vi "Configuration Window.vi"(8 "error in (no error)":errorcluster, 11 "Inst.FP":refnum<class "Inst.FP.lvclass">) -> (0 "error out":errorcluster, 3 "Inst.FP":refnum<class "Inst.FP.lvclass">)   [LabVIEW 2019, in "Inst.FP.lvclass"]
uses:
  Inst.FP.lvclass
  Typedefs/Inst.FP.Type--Enum.ctl
  Inst.FP.lvclass/Inst.FP.ctl
  FP-TC-Shared/FP-TC-Shared.lvclass
panel:
  in  "Paths":string
  in  "FP Type":T1
  in  "Cancel":bool
  in  "OK":bool
  # "Confirm or Make Changes:"
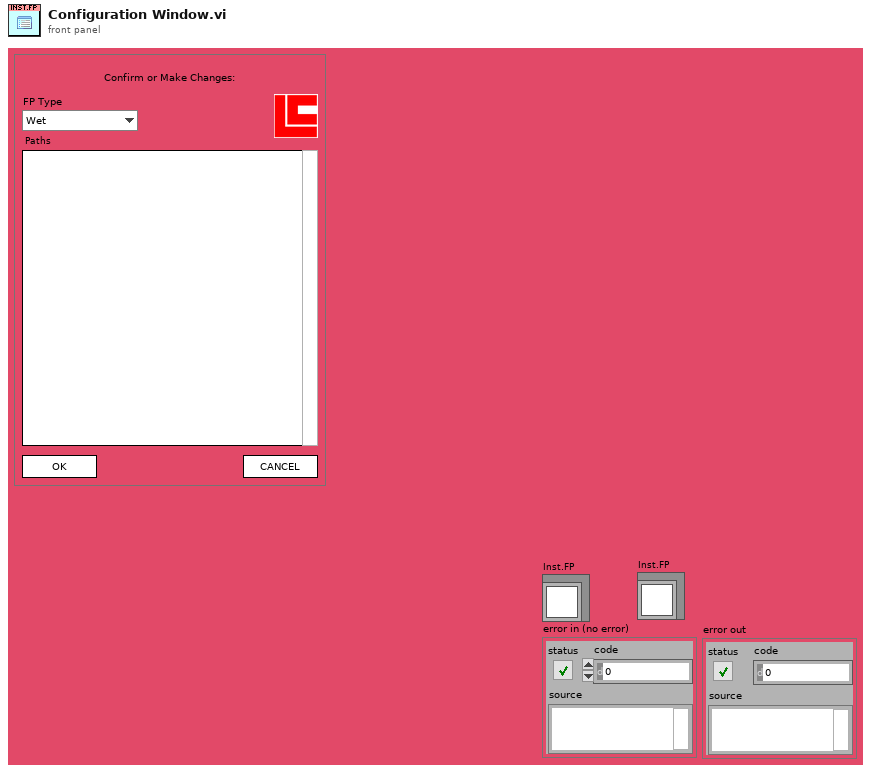
[diagram p1: front panel]
types:
  T1 = typedef "Inst.FP.lvclass/Inst.FP.Type--Enum.ctl" = enum32{"Wet", "CF"}
  T2 = enum32{"Invalid", "Standard", "Closed", "Hidden", "Minimized", "Maximized"}
  T3 = enum32{"invalid app kind", "Development System", "Run Time System", "Student Edition", "Embedded LabVIEW", "Evaluation", "Custom"}
  T4 = cluster{"Core":cluster{"Current VI Reference":refnum<vi>, "Close Panel on Exit?":bool}, "Inst.FP":refnum<class "Inst.FP.lvclass">}
  T5 = cluster{"Current VI Reference":refnum<vi>, "Close Panel on Exit?":bool}
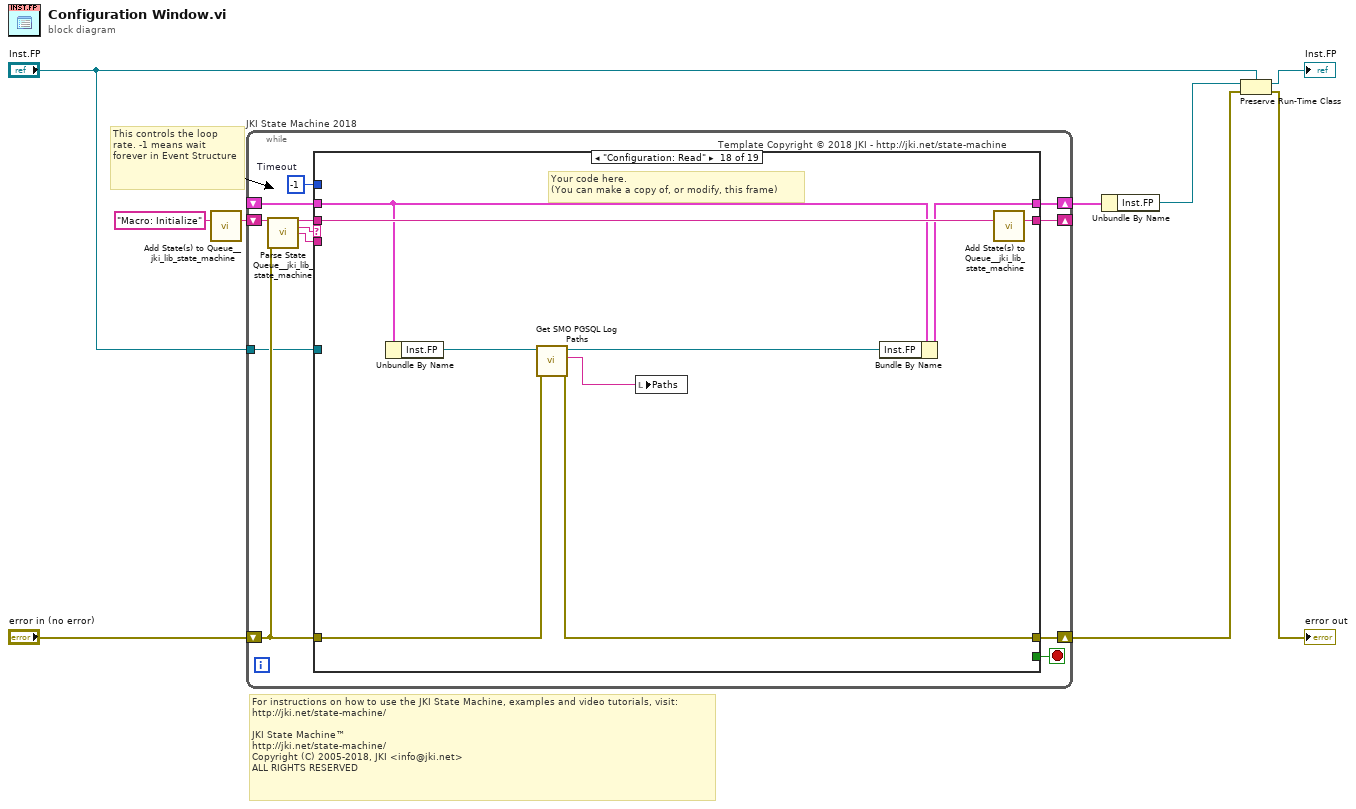
[diagram p0: block diagram]
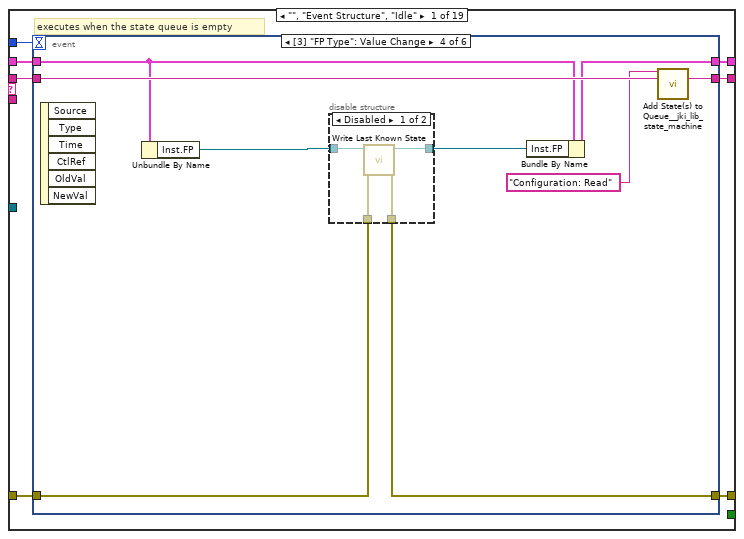
[diagram p2: hidden frame]
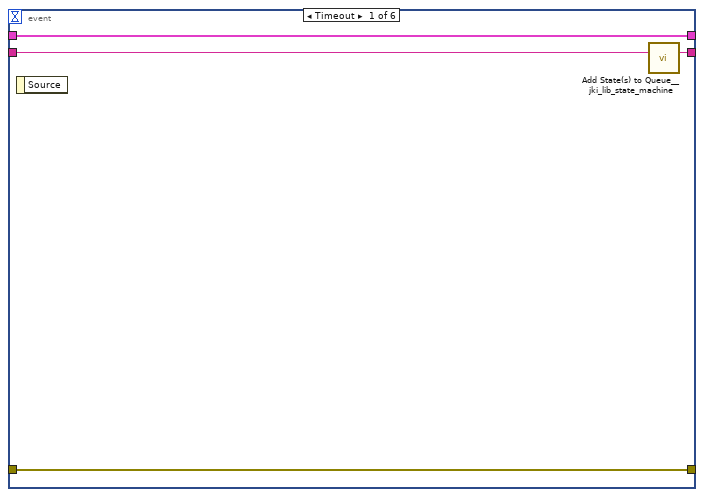
[diagram p3: hidden frame]
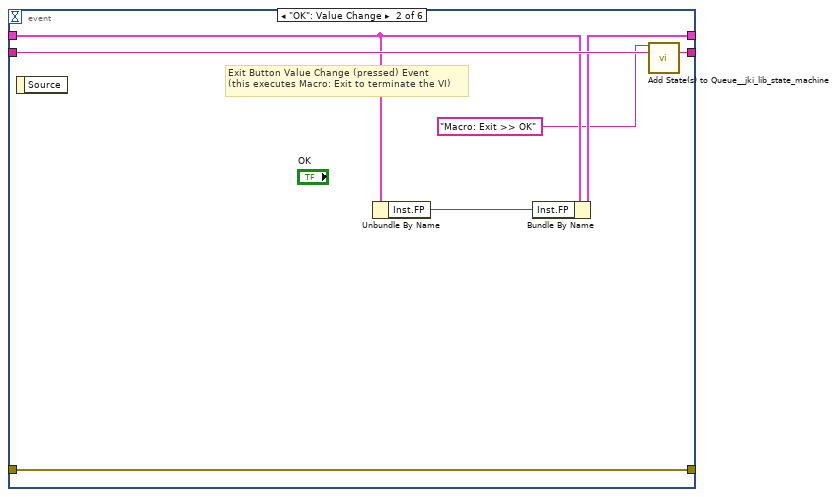
[diagram p4: hidden frame]
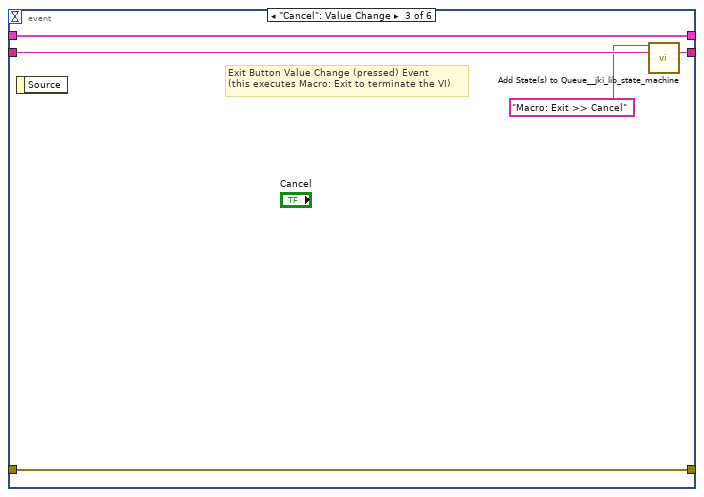
[diagram p5: hidden frame]
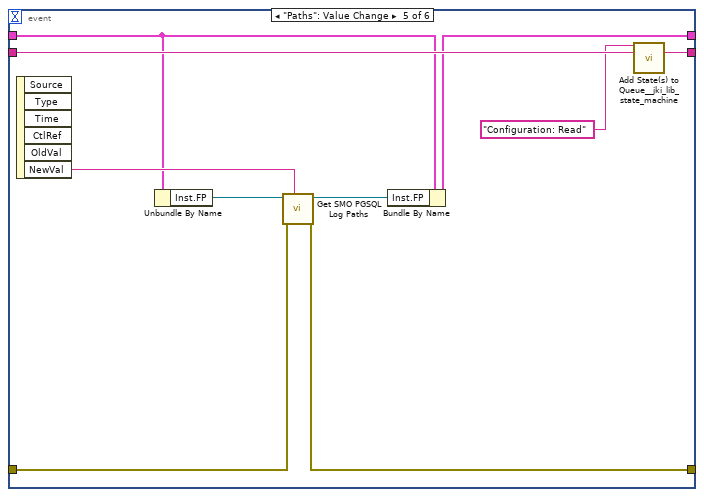
[diagram p7: hidden frame]
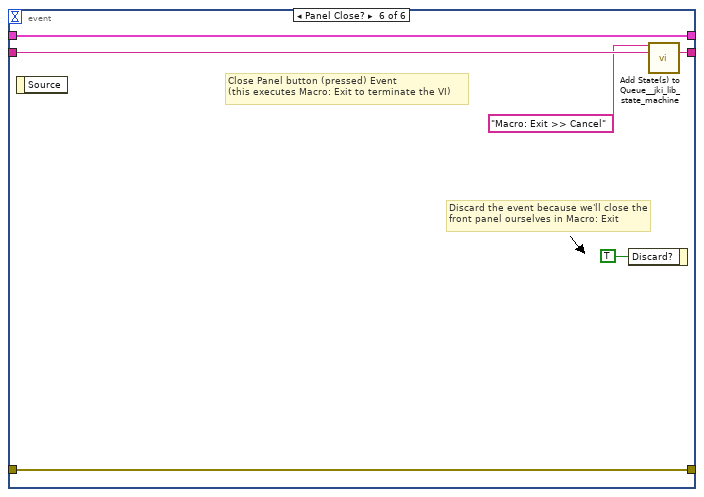
[diagram p8: hidden frame]
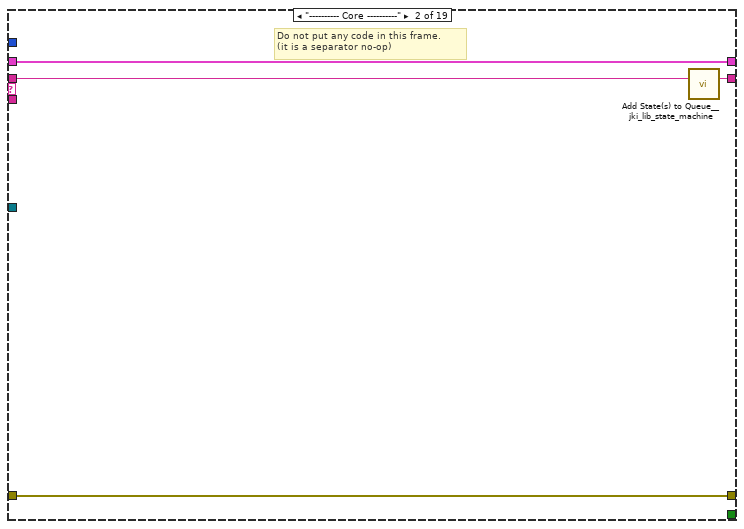
[diagram p9: hidden frame]
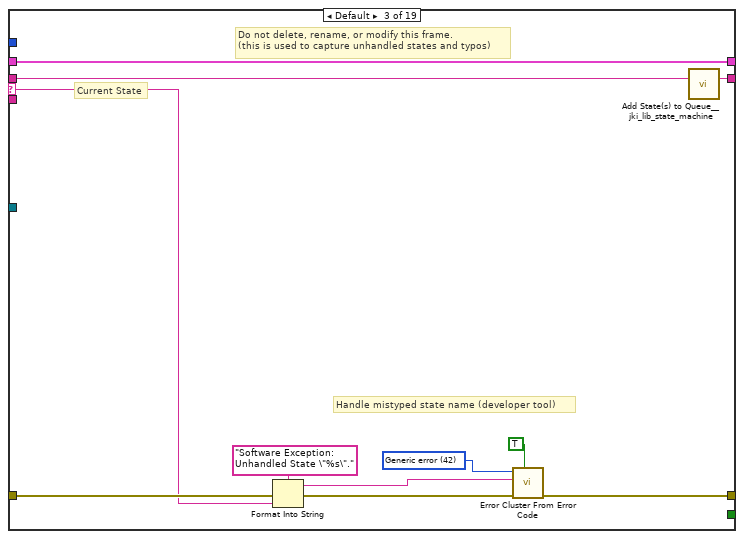
[diagram p10: hidden frame]
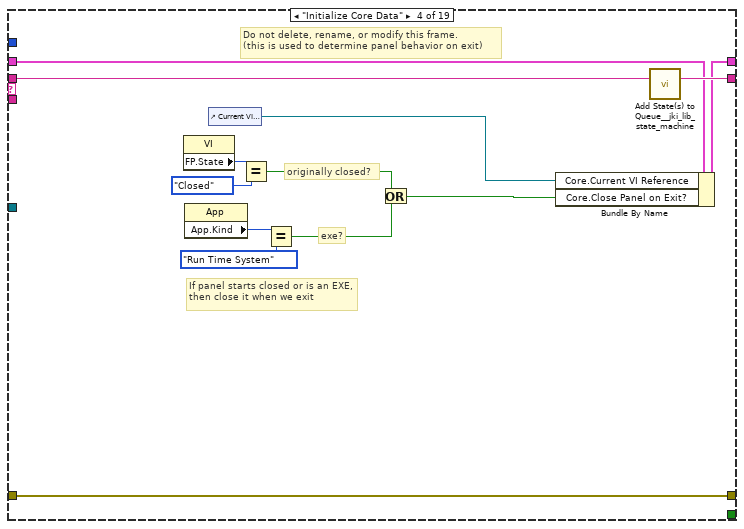
[diagram p11: hidden frame]
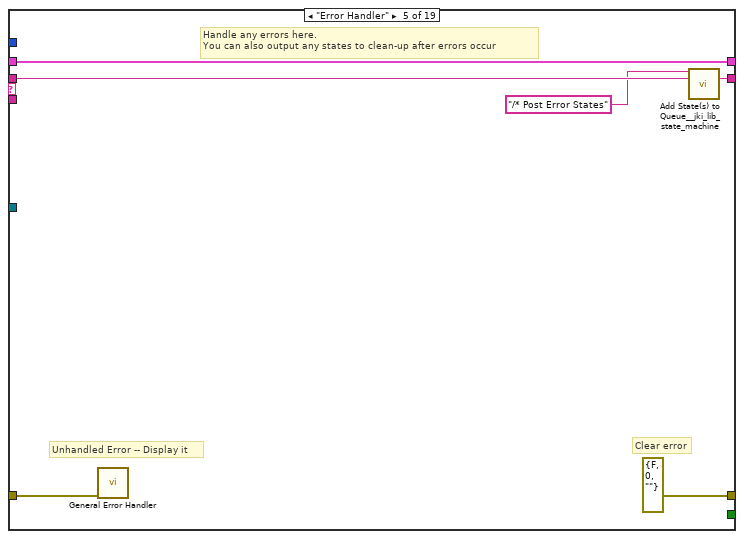
[diagram p12: hidden frame]
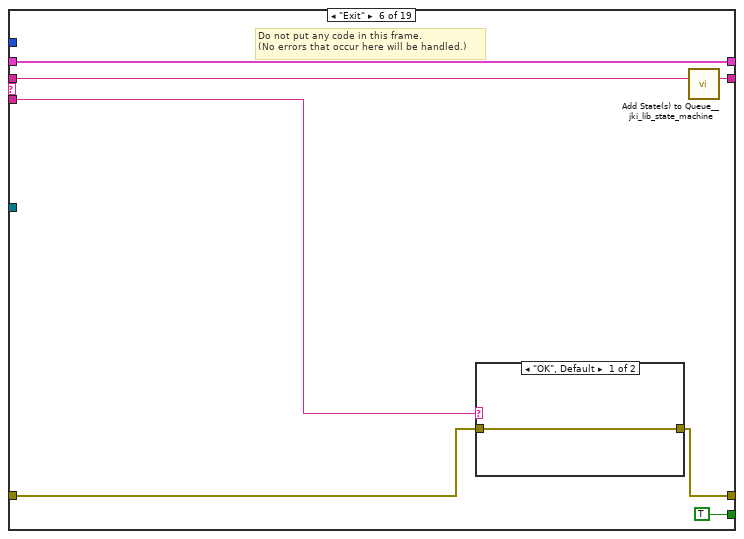
[diagram p13: hidden frame]
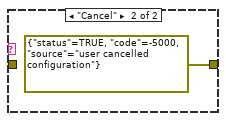
[diagram p14: hidden frame]
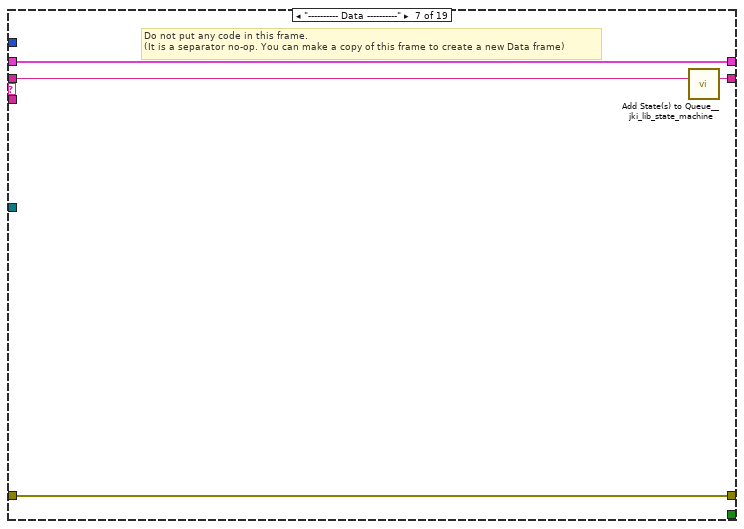
[diagram p15: hidden frame]
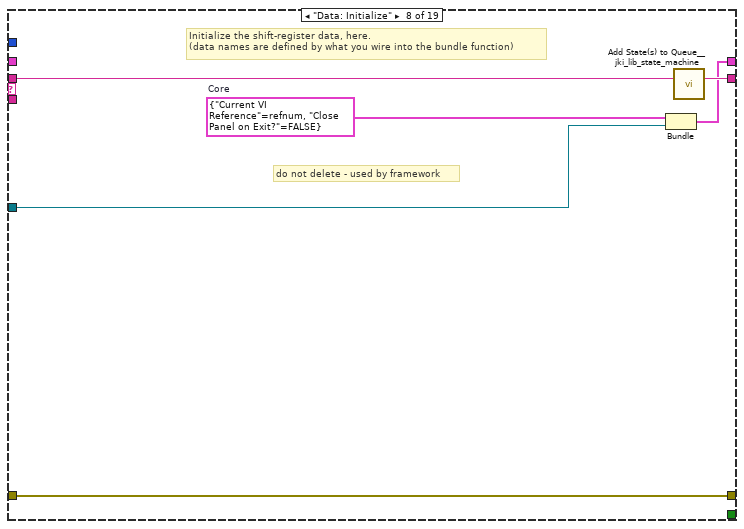
[diagram p16: hidden frame]
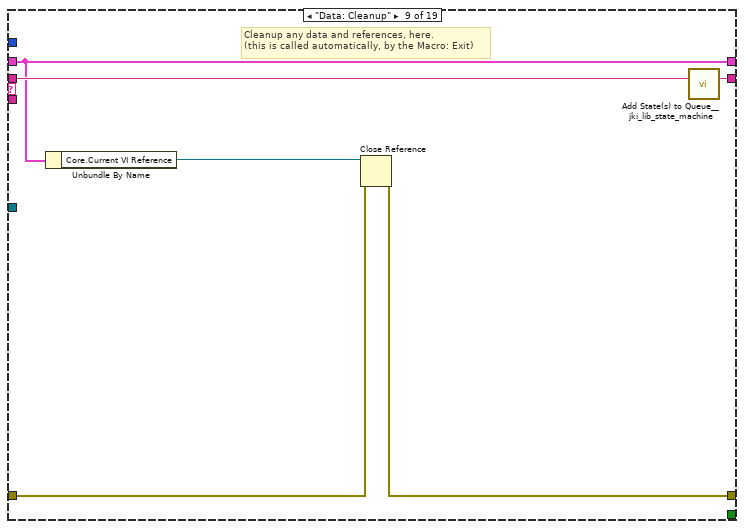
[diagram p17: hidden frame]
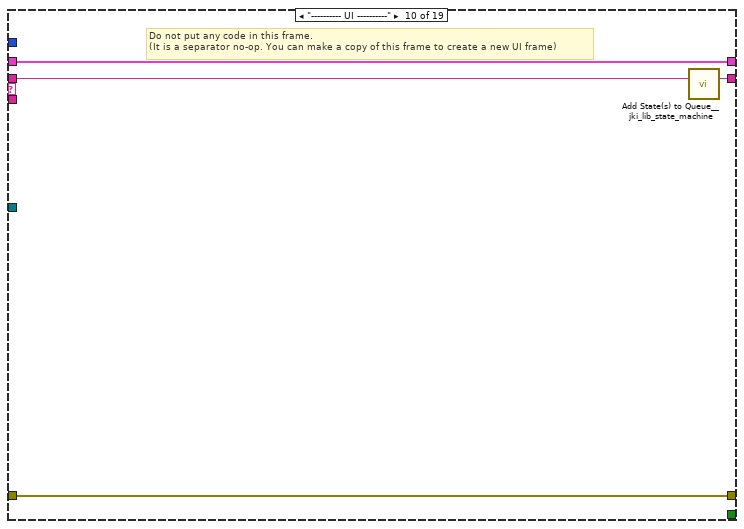
[diagram p18: hidden frame]
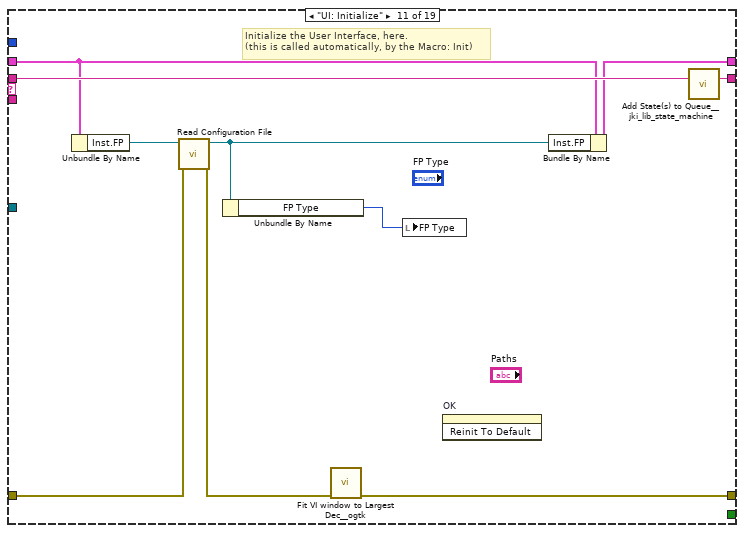
[diagram p19: hidden frame]
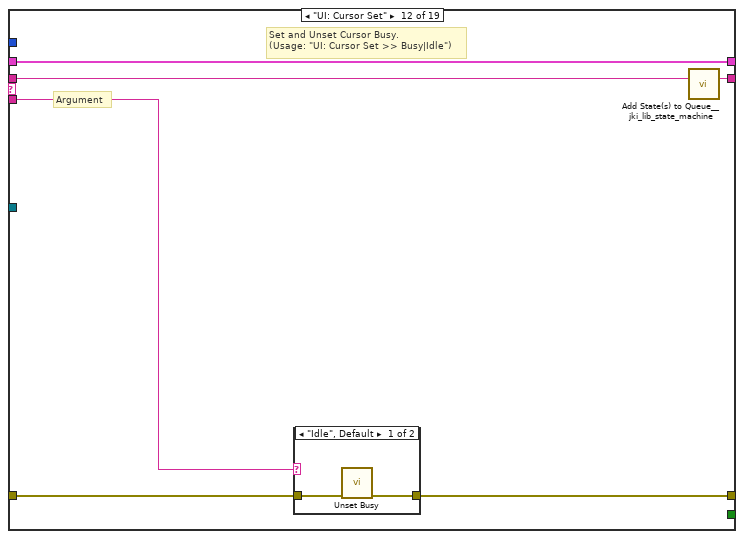
[diagram p20: hidden frame]
diagram:
  # "For instructions on how to use the JKI State Machine, examples and video tutorials, visit:\nhttp://jki.net/state-machine/\n\nJKI State Machine™\nhttp://jki.net/state-machine/\nCopyright (C) 2005-2018, JKI <info@jki.net>\nALL RIGHTS RESERVED"
  # "This controls the loop rate. -1 means wait forever in Event Structure"
  n1 = call <vilib>:"Add State(s) to Queue__jki_lib_state_machine.vi"("State(s) in (\"\")"="Macro: Initialize") -> ("States Out"=w6:string)  [unwired: 14 in]
  n2 = while "JKI State Machine 2018" {
    shift-right: [w14] -> w3
    shift-left: _ -> [w13]
    shift-right: [w17] -> w4
    shift-left: "error in (no error)" -> [w11]
    shift-right: [w16] -> _
    shift-left: w6 -> [w18]
    tunnel: "Inst.FP" -> [w10]
    stop <- w15 stop-if-true
    w12 = -1  # Timeout
    # "Template Copyright © 2018 JKI - http://jki.net/state-machine"
    n3 = call <vilib>:"Parse State Queue__jki_lib_state_machine.vi"("State Queue"=w18, "Error In (no error)"=w11) -> ("Remaining States"=w20:string, "Current State"=w21:string, "Arguments"=w19:string)  [unwired: 11 in]
    n4 = case shown="\"Configuration: Read\"" w21 {
      selector: w21 -> [_ _ w79 _ _ _ _ _ _ _ _ _ _ _ _ _ _ _ _]
      tunnel: w20 -> [w28 w78 w83 w102 w108 w115 w121 w127 w133 w137 w147 w153 w164 w233 w238 w253 w257 w266 w272]
      tunnel: w19 -> [_ _ _ _ _ w111 _ _ _ _ _ w148 w158 _ _ w242 _ _ _]
      tunnel: w13 -> [w26 w75 w81 w95 w105 w113 w118 _ w128 w134 w144 w151 w160 w230 w235 w250 w254 w263 w268]
      tunnel: [w25 w76 w85 w99 errorcluster {"status"=FALSE, "code"=0, "source"=""} ("error out") w109 w119 w123 w129 w135 w145 w149 w161 w231 w236 w251 w255 w261 w269] -> w17
      tunnel: w11 -> [w24 w76 w84 w99 w104 w110 w119 w123 w130 w135 w141 w150 w162 w231 w236 w251 w255 w262 w269]
      tunnel: [w27 w77 w82 w101 w107 w114 w120 w126 w132 w136 w146 w152 w163 w232 w237 w252 w256 w265 w271] -> w16
      tunnel: [_ _ _ _ _ TRUE _ _ _ _ _ _ _ _ _ _ _ _ _] -> w15
      tunnel: [w23 w75 w81 w100 w105 w113 w118 w125 w128 w134 w143 w151 w160 w230 w235 w250 w254 w264 w270] -> w14
      tunnel: w12 -> [w22 _ _ _ _ _ _ _ _ _ _ _ _ _ _ _ _ _ _]
      tunnel: w10 -> [_ _ _ _ _ _ _ w122 _ _ _ _ _ _ _ _ _ _ _]
      frame "", "Event Structure", "Idle" {
        # "executes when the state queue is empty"
        n5 = event shown="[3] \"FP Type\": Value Change" {
          selector: _ -> [_ _ _ _ _ _]
          dyn-events: _ -> [_ _ _ _ _ _]
          timeout: w22 -> [_ _ _ _ _ _]
          tunnel: w28 -> [w32 w39 w44 w52 w67 w74]
          tunnel: [w31 w38 w43 w53 w68 w73] -> w27
          tunnel: w26 -> [w29 w35 w40 w49 w59 w71]
          tunnel: [w30 w37 w42 w47 w63 w72] -> w25
          tunnel: w24 -> [w30 w37 w42 w48 w62 w72]
          tunnel: [w29 w36 w40 w50 w60 w71] -> w23
          event Timeout {
            n6 = event-data() -> ()  [unwired: 1 in, 1 out]
            n7 = call <vilib>:"Add State(s) to Queue__jki_lib_state_machine.vi"("State(s) in (\"\")"=w32) -> ("States Out"=w31:string)  [unwired: 14 in]
          }
          event "OK": Value Change {
            # "Exit Button Value Change (pressed) Event\n(this executes Macro: Exit to terminate the VI)"
            n8 = event-data() -> ()  [unwired: 1 in, 1 out]
            n9 = Unbundle By Name(w35) -> ("Inst.FP"=w33:refnum<class "Inst.FP.lvclass">)
            n10 = Bundle By Name(cluster=w35, "Inst.FP"=w33) -> (w36:T4)
            n11 = call <vilib>:"Add State(s) to Queue__jki_lib_state_machine.vi"("State(s) in Front (\"\")"="Macro: Exit >> OK", "State(s) in (\"\")"=w39) -> ("States Out"=w38:string)  [unwired: 13 in]
          }
          event "Cancel": Value Change {
            # "Exit Button Value Change (pressed) Event\n(this executes Macro: Exit to terminate the VI)"
            n12 = event-data() -> ()  [unwired: 1 in, 1 out]
            n13 = call <vilib>:"Add State(s) to Queue__jki_lib_state_machine.vi"("State(s) in Front (\"\")"="Macro: Exit >> Cancel", "State(s) in (\"\")"=w44) -> ("States Out"=w43:string)  [unwired: 13 in]
          }
          event Value Change {
            n14 = event-data() -> ()  [unwired: 1 in, 6 out]
            n15 = Unbundle By Name(w49) -> ("Inst.FP"=w45:refnum<class "Inst.FP.lvclass">)
            n16 = disable-structure shown="Disabled" {
              disable-tunnel: w48 -> [w57 _]
              disable-tunnel: [w56 _] -> w47
              disable-tunnel: [w55 w58] -> w46
              disable-tunnel: w45 -> [w54 w58]
              frame Disabled {
                n17 = call "Write Last Known State.vi"("error in (no error)"=w57, "FP-TC-Shared in"=w54) -> ("error out"=w56:errorcluster, "FP-TC-Shared out"=w55:refnum<class "FP-TC-Shared.lvclass">)  [unwired: 8 in]
              }
              frame Enabled {
              }
            }
            n18 = Bundle By Name(cluster=w49, "Inst.FP"=w46) -> (w50:T4)
            n19 = call <vilib>:"Add State(s) to Queue__jki_lib_state_machine.vi"("State(s) in Front (\"\")"="Configuration: Read" ("State(s) in Front (\"\")"), "State(s) in (\"\")"=w52) -> ("States Out"=w53:string)  [unwired: 13 in]
          }
          event "Paths": Value Change {
            n20 = event-data() -> ("NewVal"=w64:string)  [unwired: 1 in, 5 out]
            n21 = Unbundle By Name(w59) -> ("Inst.FP"=w65:refnum<class "Inst.FP.lvclass">)
            n22 = call-dynamic "Get SMO PGSQL Log Paths.vi"("Paths"=w64, "error in (no error)"=w62, "Inst.FP in"=w65) -> ("error out"=w63:errorcluster, "Inst.FP out"=w61:refnum<class "Inst.FP.lvclass">)  [unwired: 6 in, 1 out]
            n23 = Bundle By Name(cluster=w59, "Inst.FP"=w61) -> (w60:T4)
            n24 = call <vilib>:"Add State(s) to Queue__jki_lib_state_machine.vi"("State(s) in Front (\"\")"="Configuration: Read" ("State(s) in Front (\"\")"), "State(s) in (\"\")"=w67) -> ("States Out"=w68:string)  [unwired: 13 in]
          }
          event Panel Close? {
            # "Discard the event because we'll close the front panel ourselves in Macro: Exit"
            # "Close Panel button (pressed) Event\n(this executes Macro: Exit to terminate the VI)"
            n25 = event-data() -> ()  [unwired: 1 in, 1 out]
            n26 = event-data("Discard?"=TRUE) -> ()  [unwired: 1 in, 1 out]
            n27 = call <vilib>:"Add State(s) to Queue__jki_lib_state_machine.vi"("State(s) in Front (\"\")"="Macro: Exit >> Cancel", "State(s) in (\"\")"=w74) -> ("States Out"=w73:string)  [unwired: 13 in]
          }
        }
      }
      frame "---------- Core ----------" {
        # "Do not put any code in this frame.\n(it is a separator no-op)"
        n28 = call <vilib>:"Add State(s) to Queue__jki_lib_state_machine.vi"("State(s) in (\"\")"=w78) -> ("States Out"=w77:string)  [unwired: 14 in]
      }
      frame Default {
        w88 = 42 items=["No error", "Argument error", "Memory is full", "Out of zone", "End of file", "File already open", "Generic file I/O error", "File not found", "File permission error", "Disk is full", "Duplicate path", "Too many files open", "System feature not enabled", "Resource file not found", "Cannot add resource", "Resource not found", "Image not found", "Image memory error", "Pen does not exist", "Config type invalid", "Config token not found", "Config parse error", "Config memory error", "Bad external code format", "Bad external code offset", "External code not present", "Null window", "Destroy window error", "Null menu", "Print aborted", "Bad print record", "Print driver error", "Windows error during printing", "Memory error during printing", "Print dialog error", "Generic print error", "Invalid device refnum", "Device not found", "Device parameter error", "Device unit error", "Cannot open device", "Device call aborted", "Generic error", "Cancelled by user", "Object ID too low", "Object ID too high", "Object not in heap", "Unknown heap", "Unknown object (invalid DefProc)", "Unknown object (DefProc not in table)", "Message out of range", "Invalid (null) method", "Unknown message", "Manager call not supported", "Bad address", "Network operation in progress", "Network operation timed out", "Connection is busy", "Network attribute not supported", "Network error", "Address in use", "System out of memory", "Connection aborted", "Connection refused", "Not connected", "Already connected", "Connection closed", "Initialization error (interapplication manager)", "Bad occurrence", "Wait on unbound occurrence handler", "Occurrence queue overflow", "Datalog type conflict", "Unused", "Unrecognized type (interapplication manager)", "Memory corrupt", "Failed to make temporary DLL", "Old CIN version", "Drag socket not found", "Failed to load drop-object", "Failed to register OLE object", "Failed to release OLE object", "Format specifier type mismatch", "Unknown format specifier", "Too few format specifiers", "Too many format specifiers", "Scan failed", "Newer CIN version", "Error converting to variant", "Runtime menu error", "Password tampered", "Variant attribute not found", "Incompatible variant data type", "Event data is not available", "Event Store is not present", "Occurrence is not found", "Event Queue is not created", "Event info is not available", "Refnum passed is NULL", "Error retrieving Class GUID", "Error retrieving CoClass GUID", "Error retrieving TypeLib GUID.", "Bad built application magic bytes.", "Specific driver is different from the specific driver associated with the Logical Name.", "There is no session opened to the class driver.", "Max Error", "MAX - Error with config objects", "MAX - Error loading configuration", "MAX - Group not supported"]
        # "Current State"
        # "Do not delete, rename, or modify this frame.\n(this is used to capture unhandled states and typos)"
        # "Handle mistyped state name (developer tool)"
        n29 = Format Into String(format string="Software Exception: Unhandled State \"%s\"." ("message"), error in=w84, w79) -> (resulting string=w87:string, error out=w86:errorcluster)  [unwired: 1 in]
        n30 = call <vilib>:"Error Cluster From Error Code.vi"("show call chain? (False)"=TRUE, "error in (no error)"=w86, "error message (\"\")"=w87, "error code (0)"=w88) -> ("error out"=w85:errorcluster)  [unwired: 5 in]
        n31 = call <vilib>:"Add State(s) to Queue__jki_lib_state_machine.vi"("State(s) in (\"\")"=w83) -> ("States Out"=w82:string)  [unwired: 14 in]
      }
      frame "Initialize Core Data" {
        # "Do not delete, rename, or modify this frame.\n(this is used to determine panel behavior on exit)"
        # "originally closed?"
        # "exe?"
        # "If panel starts closed or is an EXE, then close it when we exit"
        n32 = property class="VI"() -> ("FP.State"=w92:T2)  [unwired: 2 in, 2 out]
        n33 = property class="App"() -> ("App.Kind"=w98:T3)  [unwired: 2 in, 2 out]
        n34 = control-ref of="Current VI Reference"() -> (w93:refnum<vi>)
        n35 = Equal?(x=w92, y=T2."Closed" ("Front Panel Window:State")) -> (x = y?=w90:bool)
        n36 = Equal?(x=w98, y=T3."Run Time System" ("Application:Kind")) -> (x = y?=w96:bool)
        n37 = Or(x=w90, y=w96) -> (x .or. y?=w94:bool)
        n38 = Bundle By Name(cluster=w95, "Core.Current VI Reference"=w93, "Core.Close Panel on Exit?"=w94) -> (w100:T4)
        n39 = call <vilib>:"Add State(s) to Queue__jki_lib_state_machine.vi"("State(s) in (\"\")"=w102) -> ("States Out"=w101:string)  [unwired: 14 in]
      }
      frame "Error Handler" {
        # "Unhandled Error -- Display it"
        # "Handle any errors here.\nYou can also output any states to clean-up after errors occur"
        # "Clear error"
        n40 = call <vilib>:"General Error Handler.vi"("error in (no error)"=w104) -> ()  [unwired: 10 in, 5 out]
        n41 = call <vilib>:"Add State(s) to Queue__jki_lib_state_machine.vi"("State(s) in Front (\"\")"="/* Post Error States", "State(s) in (\"\")"=w108) -> ("States Out"=w107:string)  [unwired: 13 in]
      }
      frame "Exit" {
        # "Do not put any code in this frame.\n(No errors that occur here will be handled.)"
        n42 = case shown="\"OK\", Default" w111 {
          tunnel: w110 -> [w116 _]
          tunnel: [w116 errorcluster {"status"=TRUE, "code"=-5000, "source"="user cancelled configuration"} ("error in (no error)")] -> w109
          frame "OK", Default {
          }
          frame "Cancel" {
          }
        }
        n43 = call <vilib>:"Add State(s) to Queue__jki_lib_state_machine.vi"("State(s) in (\"\")"=w115) -> ("States Out"=w114:string)  [unwired: 14 in]
      }
      frame "---------- Data ----------" {
        # "Do not put any code in this frame.\n(It is a separator no-op. You can make a copy of this frame to create a new Data frame)"
        n44 = call <vilib>:"Add State(s) to Queue__jki_lib_state_machine.vi"("State(s) in (\"\")"=w121) -> ("States Out"=w120:string)  [unwired: 14 in]
      }
      frame "Data: Initialize" {
        w124 = T5 {"Current VI Reference"=refnum, "Close Panel on Exit?"=FALSE}  # Core
        # "do not delete - used by framework"
        # "Initialize the shift-register data, here.\n(data names are defined by what you wire into the bundle function)"
        n45 = Bundle("Core"=w124, "Inst.FP"=w122) -> (w125:T4)  [unwired: 1 in]
        n46 = call <vilib>:"Add State(s) to Queue__jki_lib_state_machine.vi"("State(s) in (\"\")"=w127) -> ("States Out"=w126:string)  [unwired: 14 in]
      }
      frame "Data: Cleanup" {
        # "Cleanup any data and references, here.\n(this is called automatically, by the Macro: Exit)"
        n47 = Unbundle By Name(w128) -> ("Core.Current VI Reference"=w131:refnum<vi>)
        n48 = Close Reference(reference=w131, error in (no error)=w130) -> (error out=w129:errorcluster)
        n49 = call <vilib>:"Add State(s) to Queue__jki_lib_state_machine.vi"("State(s) in (\"\")"=w133) -> ("States Out"=w132:string)  [unwired: 14 in]
      }
      frame "---------- UI ----------" {
        # "Do not put any code in this frame.\n(It is a separator no-op. You can make a copy of this frame to create a new UI frame)"
        n50 = call <vilib>:"Add State(s) to Queue__jki_lib_state_machine.vi"("State(s) in (\"\")"=w137) -> ("States Out"=w136:string)  [unwired: 14 in]
      }
      frame "UI: Initialize" {
        # "Initialize the User Interface, here.\n(this is called automatically, by the Macro: Init)"
        n51 = Unbundle By Name(w144) -> ("Inst.FP"=w140:refnum<class "Inst.FP.lvclass">)
        n52 = call-dynamic "Read Configuration File.vi"("error in (no error)"=w141, "Inst.FP in"=w140) -> ("error out"=w142:errorcluster, "Inst.FP out"=w139:refnum<class "Inst.FP.lvclass">)  [unwired: 8 in]
        n53 = Unbundle By Name(w139) -> ("FP Type"=w138:T1)
        n54 = call <userlib>:"Fit VI window to Largest Dec__ogtk.vi"("error in (no error)"=w142) -> ("error out"=w145:errorcluster)  [unwired: 5 in, 1 out]
        n55 = local write "FP Type"(w138) -> ()
        n56 = invoke on="OK" class="Bool" method="Reinit To Default"() -> ()  [unwired: 3 in, 3 out]
        n57 = Bundle By Name(cluster=w144, "Inst.FP"=w139) -> (w143:T4)
        n58 = call <vilib>:"Add State(s) to Queue__jki_lib_state_machine.vi"("State(s) in (\"\")"=w147) -> ("States Out"=w146:string)  [unwired: 14 in]
      }
      frame "UI: Cursor Set" {
        # "Argument"
        # "Set and Unset Cursor Busy.\n(Usage: \"UI: Cursor Set >> Busy|Idle\")"
        n59 = case shown="\"Idle\", Default" w148 {
          tunnel: w150 -> [w155 w157]
          tunnel: [w154 w156] -> w149
          frame "Idle", Default {
            n60 = call <vilib>:"Unset Busy.vi"("error in (no error)"=w155) -> ("error out"=w154:errorcluster)  [unwired: 10 in]
          }
          frame "Busy" {
            n61 = call <vilib>:"Set Busy.vi"("error in (no error)"=w157) -> ("error out"=w156:errorcluster)  [unwired: 9 in, 1 out]
          }
        }
        n62 = call <vilib>:"Add State(s) to Queue__jki_lib_state_machine.vi"("State(s) in (\"\")"=w153) -> ("States Out"=w152:string)  [unwired: 14 in]
      }
      frame "UI: Front Panel State" {
        # "Argument"
        # "Set Front Panel Open or Closed\n(Usage: \"UI: Front Panel State >> Open|Close\")"
        n63 = Unbundle By Name(w160) -> ("Core.Current VI Reference"=w159:refnum<vi>)
        n64 = case shown="\"Open\", \"Standard\", Default" w158 {
          tunnel: w162 -> [w170 w185 w196 w209 w222]
          tunnel: [w172 w186 w198 w211 w224] -> w161
          tunnel: w159 -> [w171 w183 w197 w210 w223]
          frame "Open", "Standard", Default {
            w165 = T2."Standard" ("State")
            n65 = property class="VI"(reference=w171, error in=w170) -> (reference out=w168:refnum<vi>, error out=w169:errorcluster, "FP.State"=w167:T2)
            n66 = Not Equal?(x=w167, y=w165) -> (x != y?=w166:bool)
            n67 = case shown="False" w166 {
              tunnel: [w176 w178] -> w172
              tunnel: w169 -> [w175 w178]
              tunnel: w168 -> [w174 _]
              tunnel: w165 -> [w173 _]
              frame True {
                n68 = invoke class="VI" method="FP.Open"(reference=w174, error in=w175, "Activate"=TRUE, "State"=w173) -> (error out=w176:errorcluster)  [unwired: 1 in, 4 out]
              }
              frame False {
              }
            }
          }
          frame "Close", "Closed" {
            n69 = property class="VI"(reference=w183, error in=w185) -> (reference out=w182:refnum<vi>, error out=w184:errorcluster, "FP.State"=w180:T2)
            n70 = Not Equal?(x=w180, y=T2."Closed" ("Front Panel Window:State")) -> (x != y?=w179:bool)
            n71 = case shown="True" w179 {
              tunnel: [w187 w190] -> w186
              tunnel: w184 -> [w187 w189]
              tunnel: w182 -> [_ w188]
              frame False {
              }
              frame True {
                n72 = invoke class="VI" method="FP.Close"(reference=w188, error in=w189) -> (error out=w190:errorcluster)  [unwired: 1 in, 2 out]
              }
            }
          }
          frame "Hidden", "Hide" {
            w191 = T2."Hidden" ("State")
            n73 = property class="VI"(reference=w197, error in=w196) -> (reference out=w194:refnum<vi>, error out=w195:errorcluster, "FP.State"=w193:T2)
            n74 = Not Equal?(x=w193, y=w191) -> (x != y?=w192:bool)
            n75 = case shown="True" w192 {
              tunnel: [w202 w203] -> w198
              tunnel: w195 -> [w201 w203]
              tunnel: w194 -> [w200 _]
              tunnel: w191 -> [w199 _]
              frame True {
                n76 = invoke class="VI" method="FP.Open"(reference=w200, error in=w201, "State"=w199) -> (error out=w202:errorcluster)  [unwired: 2 in, 4 out]
              }
              frame False {
              }
            }
          }
          frame "Minimize", "Minimized" {
            w204 = T2."Minimized" ("State")
            n77 = property class="VI"(reference=w210, error in=w209) -> (reference out=w207:refnum<vi>, error out=w208:errorcluster, "FP.State"=w206:T2)
            n78 = Not Equal?(x=w206, y=w204) -> (x != y?=w205:bool)
            n79 = case shown="True" w205 {
              tunnel: [w215 w216] -> w211
              tunnel: w208 -> [w214 w216]
              tunnel: w207 -> [w213 _]
              tunnel: w204 -> [w212 _]
              frame True {
                n80 = invoke class="VI" method="FP.Open"(reference=w213, error in=w214, "State"=w212) -> (error out=w215:errorcluster)  [unwired: 2 in, 4 out]
              }
              frame False {
              }
            }
          }
          frame "Maximize", "Maximized" {
            w217 = T2."Maximized" ("State")
            n81 = property class="VI"(reference=w223, error in=w222) -> (reference out=w220:refnum<vi>, error out=w221:errorcluster, "FP.State"=w219:T2)
            n82 = Not Equal?(x=w219, y=w217) -> (x != y?=w218:bool)
            n83 = case shown="True" w218 {
              tunnel: [w228 w229] -> w224
              tunnel: w221 -> [w227 w229]
              tunnel: w220 -> [w226 _]
              tunnel: w217 -> [w225 _]
              frame True {
                n84 = invoke class="VI" method="FP.Open"(reference=w226, error in=w227, "State"=w225) -> (error out=w228:errorcluster)  [unwired: 2 in, 4 out]
              }
              frame False {
              }
            }
          }
        }
        n85 = call <vilib>:"Add State(s) to Queue__jki_lib_state_machine.vi"("State(s) in (\"\")"=w164) -> ("States Out"=w163:string)  [unwired: 14 in]
      }
      frame "---------- Macro ----------" {
        # "Do not put any code in this frame.\n(It is a separator no-op. You can make a copy of this frame to create a new Macro frame)"
        n86 = call <vilib>:"Add State(s) to Queue__jki_lib_state_machine.vi"("State(s) in (\"\")"=w233) -> ("States Out"=w232:string)  [unwired: 14 in]
      }
      frame "Macro: Initialize" {
        w234 = "Data: Initialize\nInitialize Core Data\nUI: Initialize\nUI: Front Panel State >> Open\nConfiguration: Read"  # Data: Initialize Initialize Core Data UI: Initialize UI: Front Panel State >> Open Configuration: Read
        # "Initialization Macro\n(This is called once, when the VI starts)"
        n87 = call <vilib>:"Add State(s) to Queue__jki_lib_state_machine.vi"("State(s) in Front (\"\")"=w234, "State(s) in (\"\")"=w238) -> ("States Out"=w237:string)  [unwired: 13 in]
      }
      frame "Macro: Exit" {
        # "Exit Macro\n(This is called once, when the VI exits)"
        n88 = Unbundle By Name(w250) -> ("Core.Close Panel on Exit?"=w249:bool)
        n89 = call <vilib>:"Build State String with Arguments__JKI_lib_State_Machine.vi"("Arguments (\"\")"=w242, "State"="Exit") -> ("State with Arguments"=w240:string)  [unwired: 4 in]
        n90 = Select(t="UI: Front Panel State >> Close", s=w249, f="") -> (s? t:f=w246:string)
        n91 = call <vilib>:"Add State(s) to Queue__jki_lib_state_machine.vi"("State(s) in Front (\"\")"="Data: Cleanup", "State(s) at Back (\"\")"=w240) -> ("States Out"=w239:string)  [unwired: 13 in]
        n92 = call <vilib>:"Add State(s) to Queue__jki_lib_state_machine.vi"("State(s) in Front (\"\")"="Configuration: Write", "State(s) in (\"\")"=w246, "State(s) at Back (\"\")"=w239) -> ("States Out"=w245:string)  [unwired: 12 in]
        n93 = call <vilib>:"Add State(s) to Queue__jki_lib_state_machine.vi"("State(s) in Front (\"\")"=w245, "State(s) in (\"\")"=w253) -> ("States Out"=w252:string)  [unwired: 13 in]
      }
      frame "---------- Configuration ----------" {
        # "Template Separator\n(You can make a copy of, or modify, this frame)"
        n94 = call <vilib>:"Add State(s) to Queue__jki_lib_state_machine.vi"("State(s) in (\"\")"=w257) -> ("States Out"=w256:string)  [unwired: 14 in]
      }
      frame "Configuration: Read" {
        # "Your code here.\n(You can make a copy of, or modify, this frame)"
        n95 = Unbundle By Name(w263) -> ("Inst.FP"=w260:refnum<class "Inst.FP.lvclass">)
        n96 = call-dynamic "Get SMO PGSQL Log Paths.vi"("error in (no error)"=w262, "Inst.FP in"=w260) -> ("error out"=w261:errorcluster, "Paths"=w258:string, "Inst.FP out"=w259:refnum<class "Inst.FP.lvclass">)  [unwired: 7 in]
        n97 = local write "Paths"(w258) -> ()
        n98 = Bundle By Name(cluster=w263, "Inst.FP"=w259) -> (w264:T4)
        n99 = call <vilib>:"Add State(s) to Queue__jki_lib_state_machine.vi"("State(s) in (\"\")"=w266) -> ("States Out"=w265:string)  [unwired: 14 in]
      }
      frame "Configuration: Write" {
        n100 = Unbundle By Name(w268) -> ("Inst.FP"=w267:refnum<class "Inst.FP.lvclass">)
        n101 = Bundle By Name(cluster=w268, "Inst.FP"=w267) -> (w270:T4)
        n102 = call <vilib>:"Add State(s) to Queue__jki_lib_state_machine.vi"("State(s) in (\"\")"=w272) -> ("States Out"=w271:string)  [unwired: 14 in]
      }
    }
  }
  n103 = Unbundle By Name(w3) -> ("Inst.FP"=w2:refnum<class "Inst.FP.lvclass">)
  n104 = Preserve Run-Time Class(object in=w2, error in=w4, 2:"Inst.FP") -> (object out=→"Inst.FP":refnum<class "Inst.FP.lvclass">, error out=→"error out":errorcluster)
